vi "automatic_resume.vi"(8 "error in (no error)":errorcluster, 11 "index":i32) -> (0 "error out":errorcluster)   [LabVIEW 2015, in "lv-recipe-machine.lvlib"]
uses:
  lv-recipe-machine.lvlib
  _controls/error.ctl
  _controls/automatic_state.ctl
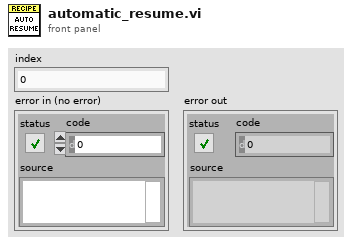
[diagram p1: front panel]
types:
  T1 = typedef "lv-recipe-machine.lvlib/error.ctl" = enum16{"<error>", "bad_command", "command_queue_timeout", "stop_notifier_timeout", "die_command_timeout", "not_in_manual_mode", "not_in_automatic_mode", "not_in_automatic_idle", "not_in_automatic_running", "not_in_automatic_paused", "automatic_step_not_found", "manual_action_not_found", "automatic_not_transition_vi", "transition_step_not_found", "unsupported_vi_type", "<null>"}
  T2 = typedef "lv-recipe-machine.lvlib/automatic_state.ctl" = enum16{"<automatic_state>", "failed", "idle", "running", "paused", "stopped", "<null>"}
  T3 = typedef "lv-recipe-machine.lvlib/references.ctl" = cluster{"semaphore":T4, "input_queue":refnum<queue>, "output_queue":refnum<queue>, "transition_queue":refnum<queue>, "data_dvr":refnum<data-value>, "stop_notifier":refnum<notifier>, "change_in_event":refnum<user-event>, "change_out_event":refnum<user-event>, "status_event":refnum<user-event>}
  T4 = typedef "Semaphore RefNum" = refnum<k1>
  T5 = typedef "lv-recipe-machine.lvlib/data.ctl" = cluster{"configuration":T6, "working":cluster{"recipe_data":T7}}
  T6 = typedef "lv-recipe-machine.lvlib/configuration.ctl" = cluster{"change_in_timeout_ms":i32}
  T7 = typedef "lv-recipe-machine.lvlib/recipe_data.ctl" = cluster{"mode":T8, "manual_state":T9, "automatic_state":T2, "previous_automatic_state":T2, "error":errorcluster, "timer []":T10[], "manual":cluster{"step_action":string, "data":variant, "actions":variant}, "automatic":cluster{"data":variant, "steps":variant, "criteria":variant, "transition":string, "index":i32, "step_launched":bool, "recipe []":T11[]}}
  T8 = typedef "lv-recipe-machine.lvlib/mode.ctl" = enum16{"<mode>", "manual", "automatic", "<null>"}
  T9 = typedef "lv-recipe-machine.lvlib/manual_state.ctl" = enum16{"<manual_state>", "failed", "action", "running", "idle", "<null>"}
  T10 = typedef "lv-recipe-machine.lvlib/timer.ctl" = cluster{"elapsed_time":dbl, "previous_time":dbl}
  T11 = typedef "lv-recipe-machine.lvlib/recipe_step.ctl" = cluster{"step":string, "data":variant}
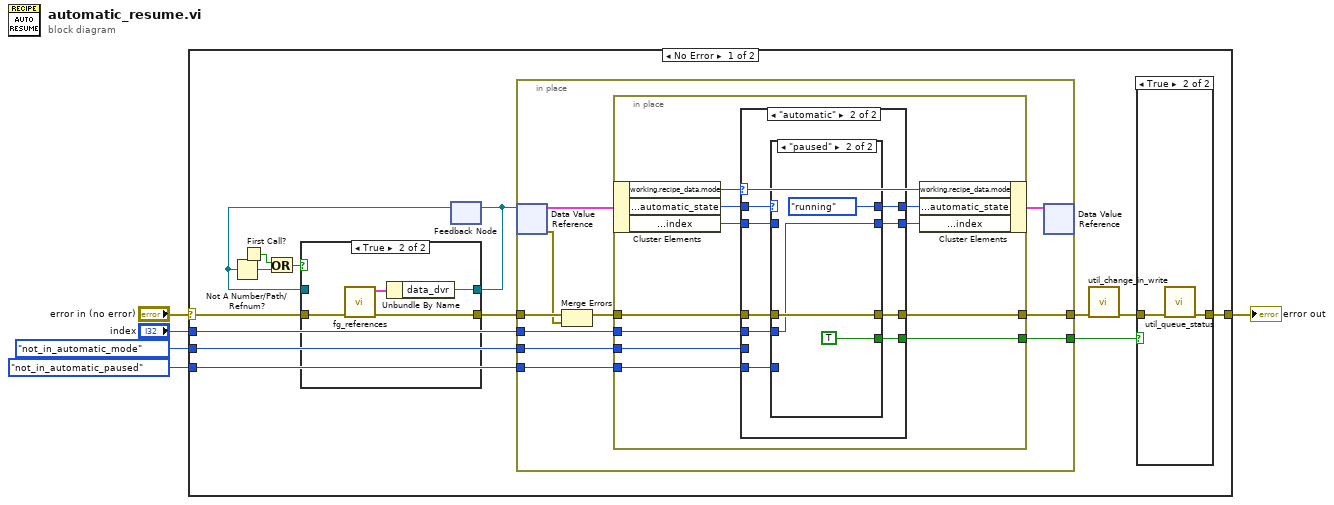
[diagram p0: block diagram]
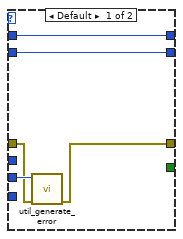
[diagram p3: hidden frame]
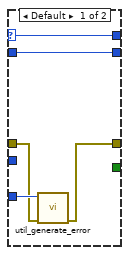
[diagram p4: hidden frame]
diagram:
  n1 = case shown="No Error" "error in (no error)" {
    selector: "error in (no error)" -> [w7 w73]
    tunnel: [w15 w73] -> w4
    tunnel: error."not_in_automatic_mode" ("error") -> [w19 _]
    tunnel: error."not_in_automatic_paused" ("error") -> [w18 _]
    tunnel: "index" -> [w6 _]
    frame No Error {
      n2 = First Call?() -> (First Call?: T/F=w12:bool)
      n3 = feedback #1() -> (w11:refnum<data-value>)  [unwired: 1 in]
      n4 = Not A Number/Path/Refnum?(number/path/refnum=w11) -> (NaN/Path/Refnum?=w13:bool)
      n5 = Or(x=w12, y=w13) -> (x .or. y?=w10:bool)
      n6 = case shown="True" w10 {
        tunnel: w7 -> [w20 w25]
        tunnel: [w20 w24] -> w8
        tunnel: [w21 w22] -> w9
        tunnel: w11 -> [w21 _]
        frame False {
        }
        frame True {
          n7 = call "fg_references.vi"("error in (no error)"=w25) -> ("error out"=w24:errorcluster, "references out"=w23:T3)  [unwired: 9 in]
          n8 = Unbundle By Name(w23) -> ("data_dvr"=w22:refnum<data-value>)
        }
      }
      n9 = feedback-in #1(w9) -> ()
      n10 = in-place {
        in-place-border: w8 -> [w35]
        in-place-border: w19 -> [w30]
        in-place-border: [w29] -> w16
        in-place-border: w18 -> [w28]
        in-place-border: [w27] -> w14
        in-place-border: w6 -> [w26]
        n11 = in-place-dvr #2(w9) -> (w33:T5, w34:errorcluster)
        n12 = Merge Errors(w35, w34) -> (w32:errorcluster)
        n13 = in-place {
          in-place-border: w32 -> [w44]
          in-place-border: w30 -> [w43]
          in-place-border: [w42] -> w29
          in-place-border: w28 -> [w38]
          in-place-border: [w37] -> w27
          in-place-border: w26 -> [w36]
          n14 = in-place-cluster #3(w33) -> ("working.recipe_data.mode"=w41:T8, "working.recipe_data.automatic_state"=w46:T2, "working.recipe_data.automatic.index"=w45:i32)
          n15 = case shown="\"automatic\"" w41 {
            tunnel: w46 -> [w48 w59]
            tunnel: w45 -> [w47 w58]
            tunnel: w44 -> [w50 w57]
            tunnel: w43 -> [w51 _]
            tunnel: [w49 w56] -> w42
            tunnel: [w48 w54] -> w40
            tunnel: [w47 w55] -> w39
            tunnel: w38 -> [_ w60]
            tunnel: [_ w53] -> w37
            tunnel: w36 -> [_ w52]
            frame Default {
              n16 = call "util_generate_error.vi"("error in (no error)"=w50, "error"=w51) -> ("error out"=w49:errorcluster)  [unwired: 9 in]
            }
            frame "automatic" {
              n17 = case shown="\"paused\"" w59 {
                selector: w59 -> [w61 _]
                tunnel: w60 -> [w65 _]
                tunnel: w58 -> [w62 _]
                tunnel: w57 -> [w64 w69]
                tunnel: [w63 w69] -> w56
                tunnel: [w62 w66] -> w55
                tunnel: [w61 automatic_state."running" ("automatic_state")] -> w54
                tunnel: [_ TRUE] -> w53
                tunnel: w52 -> [_ w66]
                frame Default {
                  n18 = call "util_generate_error.vi"("error in (no error)"=w64, "error"=w65) -> ("error out"=w63:errorcluster)  [unwired: 9 in]
                }
                frame "paused" {
                }
              }
            }
          }
          n19 = in-place-cluster #3("working.recipe_data.mode"=w41, "working.recipe_data.automatic_state"=w40, "working.recipe_data.automatic.index"=w39) -> (w31:T5)
        }
        n20 = in-place-dvr #2(w31) -> ()  [unwired: 2 out]
      }
      n21 = call "util_change_in_write.vi"("error in (no error)"=w16) -> ("error out"=w17:errorcluster)  [unwired: 10 in]
      n22 = case shown="True" w14 {
        tunnel: w17 -> [w70 w72]
        tunnel: [w70 w71] -> w15
        frame False {
        }
        frame True {
          n23 = call "util_queue_status.vi"("error in (no error)"=w72) -> ("error out"=w71:errorcluster)  [unwired: 10 in]
        }
      }
    }
    frame Error {
    }
  }
  "error out" <- w4
